vi "UI.Connection.State.Get.vi"(6 "Menu Ref":refnum<k9>, 7 "Name Ref":refnum<vi>, 8 "error in (no error)":errorcluster, 9 "Addon Path in":string, 10 "NIVS.System Definition Root in":refnum<k24>, 11 "NIVS.Workspace Ref in":T1) -> (0 "error out":errorcluster, 1 "Addon Connected?":bool, 2 "NIVS.System Definition Root out":refnum<k24>, 3 "NIVS.Workspace Ref out":T1, 5 "NIVS.SysDef Ref out":refnum<k24>)   [LabVIEW 2019, in "Control Workspace Shared.lvlib"]
uses:
  Control Workspace Shared.lvlib
  <vilib>/NI VeriStand/Execution/Workspace/WorkspaceAPI.ctl
  NationalInstruments.VeriStand.ClientAPI
  <vilib>/NI VeriStand/Execution/Workspace/NI_VS Workspace ExecutionAPI.lvlib
  NationalInstruments.VeriStand.SystemDefinitionAPI
  NationalInstruments.VeriStand.SystemStorage
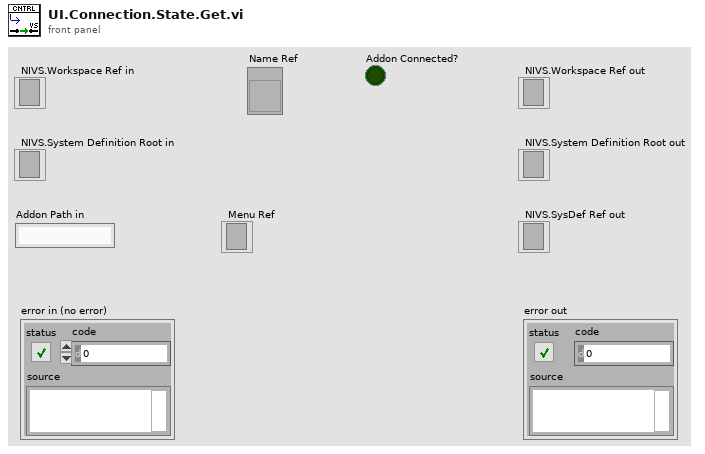
[diagram p1: front panel]
types:
  T1 = typedef "NI_VS Workspace ExecutionAPI.lvlib/WorkspaceAPI.ctl" = refnum<k24>
  T2 = typedef "NI_VS Workspace ExecutionAPI.lvlib/SystemState.ctl" = u8
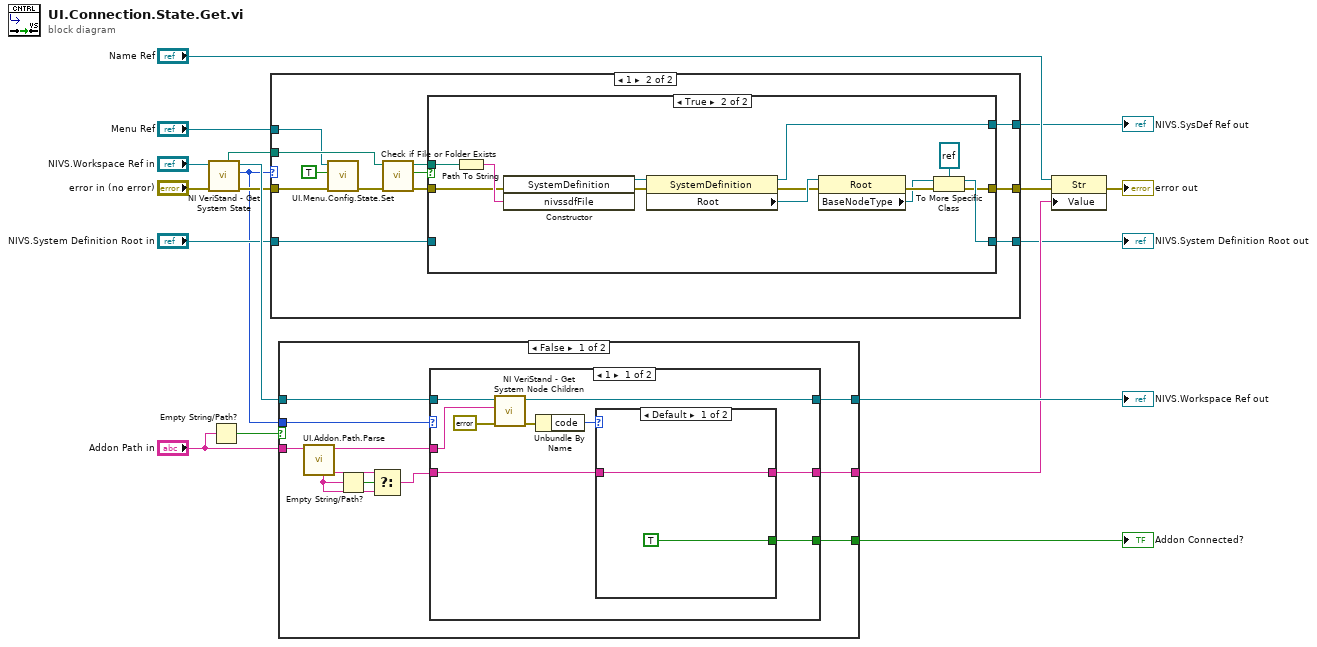
[diagram p0: block diagram]
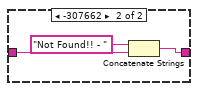
[diagram p2: hidden frame]
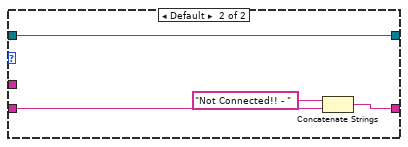
[diagram p3: hidden frame]
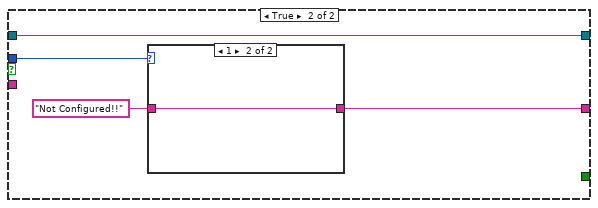
[diagram p4: hidden frame]
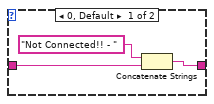
[diagram p5: hidden frame]
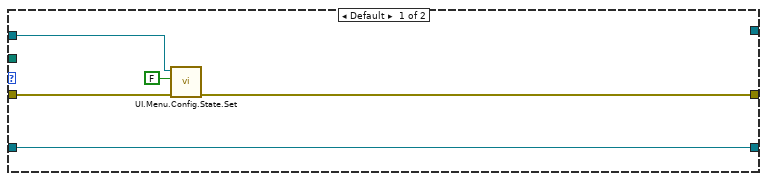
[diagram p6: hidden frame]
diagram:
  n1 = call <vilib>:"NI VeriStand - Get System State.vi"("error in (no error)"="error in (no error)", "WorkspaceManager in"="NIVS.Workspace Ref in") -> ("error out"=w7:errorcluster, "System State"=w4:T2, "WorkspaceManager  out"=w9:T1, "System Definition File"=w6:path)  [unwired: 5 in, 1 out]
  n2 = Empty String/Path?(string/path="Addon Path in") -> (empty?=w15:bool)
  n3 = case shown="1" w4 {
    tunnel: [w23 w35] -> w2
    tunnel: [w21 w34] -> w5
    tunnel: "NIVS.System Definition Root in" -> [w23 w31]
    tunnel: w7 -> [w20 w26]
    tunnel: w6 -> [_ w30]
    tunnel: "Menu Ref" -> [w19 w25]
    tunnel: [_ w24] -> w1
    frame Default {
      n4 = call "UI.Menu.Config.State.Set.vi"("error in (no error)"=w20, "Enabled"=FALSE, "menu reference"=w19) -> ("error out"=w21:errorcluster)  [unwired: 8 in]
    }
    frame 1 {
      n5 = call "UI.Menu.Config.State.Set.vi"("error in (no error)"=w26, "Enabled"=TRUE, "menu reference"=w25) -> ("error out"=w27:errorcluster)  [unwired: 8 in]
      n6 = call <vilib>:"Check if File or Folder Exists.vi"("error in (no error)"=w27, "path"=w30) -> ("error out"=w33:errorcluster, "file or folder exists?"=w32:bool, "dup path"=w29:path)  [unwired: 7 in]
      n7 = case shown="True" w32 {
        tunnel: [w36 w40] -> w35
        tunnel: [w37 w39] -> w34
        tunnel: w33 -> [w37 w47]
        tunnel: w29 -> [_ w46]
        tunnel: w31 -> [w36 _]
        tunnel: [_ w38] -> w24
        frame False {
        }
        frame True {
          n8 = Path To String(path=w46) -> (string=w49:string)
          n9 = constructor class="SystemDefinition"(error in=w47, "nivssdfFile"=w49) -> (reference out=w50:refnum<k24>, error out=w48:errorcluster)  [unwired: 2 in, 2 out]
          n10 = property class="SystemDefinition"(reference=w50, error in=w48) -> (reference out=w38:refnum<k24>, error out=w41:errorcluster, "Root"=w42:refnum<k24>)
          n11 = property class="Root"(reference=w42, error in=w41) -> (error out=w45:errorcluster, "BaseNodeType"=w44:refnum<k24>)  [unwired: 1 out]
          n12 = To More Specific Class(target class=refnum<k24> refnum, reference=w44, error in=w45) -> (specific class reference=w40:refnum<k24>, error out=w39:errorcluster)
        }
      }
    }
  }
  "NIVS.System Definition Root out" <- w2
  "NIVS.SysDef Ref out" <- w1
  n13 = case shown="False" w15 {
    tunnel: [w61 w80] -> w13
    tunnel: [w60 w83] -> w18
    tunnel: "Addon Path in" -> [w56 _]
    tunnel: [w59 _] -> w14
    tunnel: w4 -> [w57 w82]
    tunnel: w9 -> [w58 w83]
    frame False {
      n14 = call "UI.Addon.Path.Parse.vi"("Cached Addon Path"=w56) -> ("Addon Name"=w52:string, "Addon Path"=w55:string, "Remaining Path"=w53:string)  [unwired: 6 in, 2 out]
      n15 = Empty String/Path?(string/path=w53) -> (empty?=w54:bool)
      n16 = Select(t=w52, s=w54, f=w53) -> (s? t:f=w51:string)
      n17 = case shown="1" w57 {
        tunnel: [w70 w79] -> w61
        tunnel: w51 -> [w69 w77]
        tunnel: [w66 w78] -> w60
        tunnel: [w65 _] -> w59
        tunnel: w58 -> [w64 w78]
        tunnel: w55 -> [w62 _]
        frame 1 {
          n18 = call <vilib>:"NI VeriStand - Get System Node Children.vi"("error in (no error)"=errorcluster {"status"=FALSE, "code"=0, "source"=""}, "Node"=w62, "WorkspaceManager in"=w64) -> ("error out"=w68:errorcluster, "WorkspaceManager out"=w66:T1)  [unwired: 6 in, 1 out]
          n19 = Unbundle By Name(w68) -> ("code"=w67:i32)
          n20 = case shown="Default" w67 {
            tunnel: w69 -> [w72 w74]
            tunnel: [w72 w75] -> w70
            tunnel: [TRUE _] -> w65
            frame Default {
            }
            frame -307662 {
              n21 = Concatenate Strings("Not Found!! - " ("string"), w74) -> (w75:string)
            }
          }
        }
        frame Default {
          n22 = Concatenate Strings("Not Connected!! - " ("string"), w77) -> (w79:string)
        }
      }
    }
    frame True {
      n23 = case shown="1" w82 {
        tunnel: [w85 w87] -> w80
        tunnel: "Not Configured!!" ("CD Path in") -> [w86 w87]
        frame 0, Default {
          n24 = Concatenate Strings("Not Connected!! - " ("string"), w86) -> (w85:string)
        }
        frame 1 {
        }
      }
    }
  }
  "NIVS.Workspace Ref out" <- w18
  "Addon Connected?" <- w14
  n25 = property class="Str"(reference="Name Ref", error in=w5, "Value"=w13) -> (error out=→"error out":errorcluster)  [unwired: 1 out]
